vi "Calculator.vi"() -> ()   [LabVIEW 2012]
panel:
  in  "evaluate":bool
  in  "stop":bool
  in  "expression":string
  out "log":string
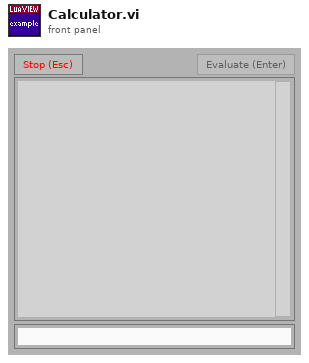
[diagram p1: front panel]
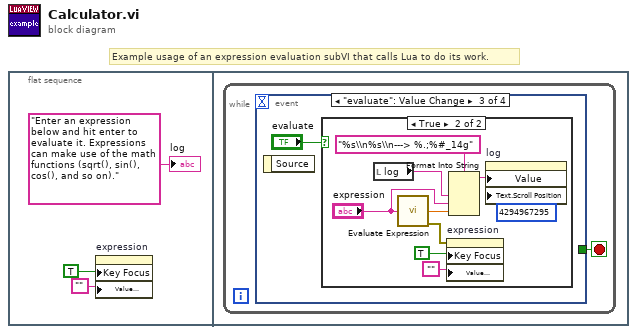
[diagram p0: block diagram]
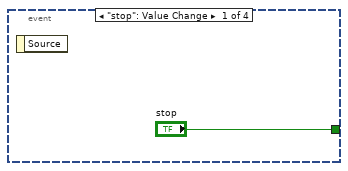
[diagram p2: hidden frame]
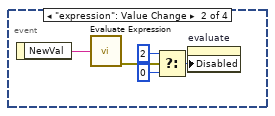
[diagram p3: hidden frame]
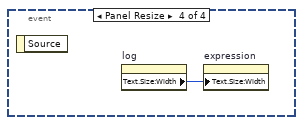
[diagram p5: hidden frame]
diagram:
  # "Example usage of an expression evaluation subVI that calls Lua to do its work."
  n1 = flat-sequence {
    frame #0 {
      n2 = property on="expression" class="Str"("Key Focus"=TRUE, "Value (Signaling)"="") -> ()  [unwired: 2 in, 2 out]
      "log" <- "Enter an expression below and hit enter to evaluate it. Expressions can make use of the math functions (sqrt(), sin(), cos(), and so on)." ("log")
    }
    frame #1 {
      n3 = while {
        stop <- w4 stop-if-true
        n4 = event shown="[2] \"evaluate\": Value Change" {
          selector: _ -> [_ _ _ _]
          dyn-events: _ -> [_ _ _ _]
          timeout: _ -> [_ _ _ _]
          tunnel: ["stop" _ _ _] -> w4
          event "stop": Value Change {
            n5 = event-data() -> ()  [unwired: 1 in, 1 out]
          }
          event "expression": Value Change {
            n6 = event-data() -> ("NewVal"=w10:string)  [unwired: 1 in]
            n7 = call "Evaluate Expression.vi"("expression"=w10) -> ("error out"=w9:errorcluster)  [unwired: 13 in, 1 out]
            n8 = Select(t=u8 2 ("Disabled"), s=w9, f=u8 0 ("Disabled")) -> (s? t:f=w8:u8)
            n9 = property on="evaluate" class="Bool"("Disabled"=w8) -> ()  [unwired: 2 in, 2 out]
          }
          event "evaluate": Value Change {
            n10 = event-data() -> ()  [unwired: 1 in, 1 out]
            n11 = case shown="True" "evaluate" {
              frame False {
              }
              frame True {
                n12 = local read "log"() -> (w17:string)
                n13 = call "Evaluate Expression.vi"("expression"="expression") -> ("result"=w19:dbl, "error out"=w15:errorcluster)  [unwired: 13 in]
                n14 = property on="expression" class="Str"(error in=w15, "Key Focus"=TRUE, "Value (Signaling)"="") -> ()  [unwired: 1 in, 2 out]
                n15 = Format Into String(format string="%s\\n%s\\n---> %.;%#_14g", w17, "expression", w19) -> (resulting string=w13:string)  [unwired: 2 in, 1 out]
                n16 = property on="log" class="Str"("Value"=w13, "Text.Scroll Position"=u32 4294967295) -> ()  [unwired: 2 in, 2 out]
              }
            }
          }
          event Panel Resize {
            n17 = event-data() -> ()  [unwired: 1 in, 1 out]
            n18 = property on="log" class="Str"() -> ("Text.Size:Width"=w21:u32)  [unwired: 2 in, 2 out]
            n19 = property on="expression" class="Str"("Text.Size:Width"=w21) -> ()  [unwired: 2 in, 2 out]
          }
        }
      }
    }
  }
